vi "pumpStop.vi"(8 "error in (no error)":errorcluster, 11 "VISA resource name":refnum<visa-resource-name>) -> (0 "error out":errorcluster)   [LabVIEW 2013]
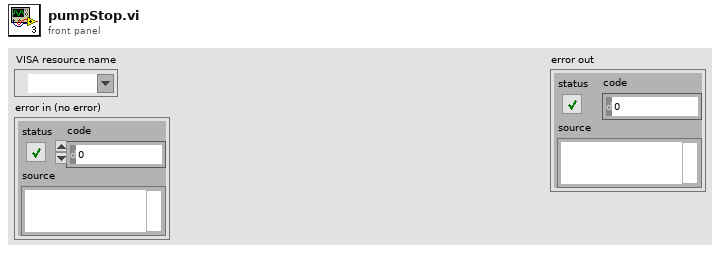
[diagram p1: front panel]
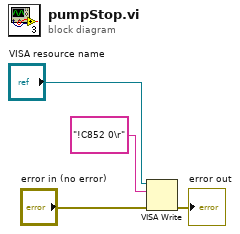
[diagram p0: block diagram]
diagram:
  n1 = VISA Write(VISA resource name="VISA resource name", write buffer="!C852 0\r" ("Command"), error in (no error)="error in (no error)") -> (error out=→"error out":errorcluster)  [unwired: 2 out]
